vi "Set SubPanel Controls Values.vi"(7 "Subpanels Map":map{string, refnum<vi>}(c390), 8 "error in (no error)":errorcluster, 11 "Schedule Block in":refnum<class "Schedule Block.lvclass">) -> (0 "error out":errorcluster, 2 "SBlock Type":string, 3 "SubPanel VI out":refnum<vi>)   [LabVIEW 2020, in "CIRCUS_uServices.lvlib" / "Scheduler.lvlib" / "Scheduler.lvclass"]
uses:
  Scheduler.lvclass
  Run Utilities/Schedule Block/Schedule Block.lvclass
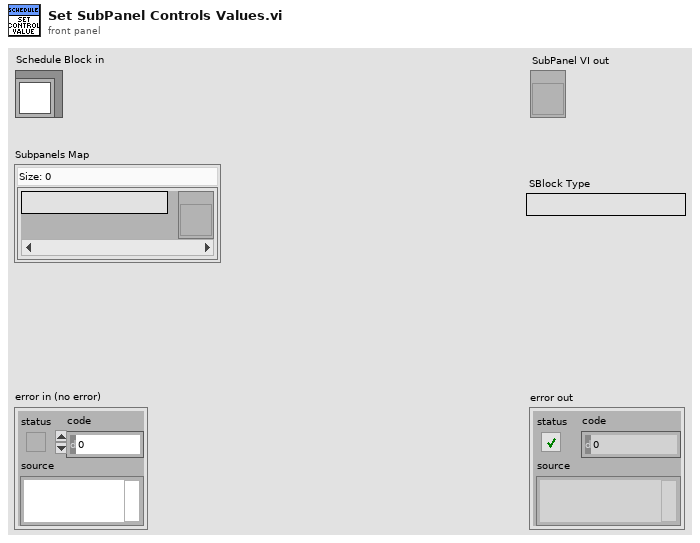
[diagram p1: front panel]
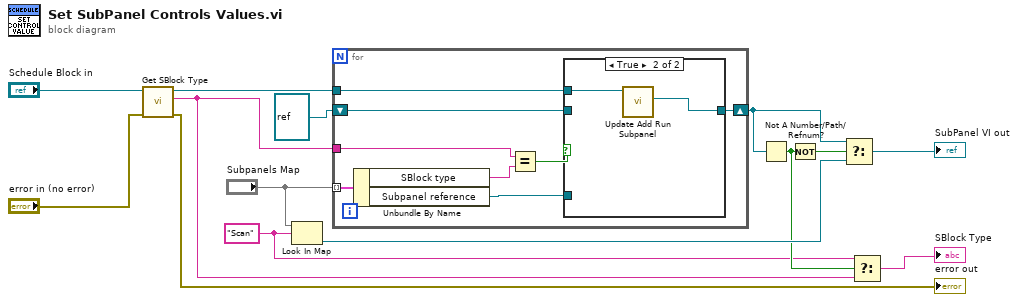
[diagram p0: block diagram]
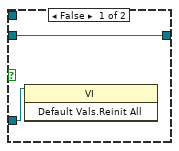
[diagram p2: hidden frame]
diagram:
  w2 = "Scan" ("f")
  n1 = call-dynamic "Get SBlock Type.vi"("error in (no error)"="error in (no error)", "Schedule Block in"="Schedule Block in") -> ("error out"=→"error out":errorcluster, "SBlock Type"=w3:string, "Schedule Block out"=w10:refnum<class "Schedule Block.lvclass">)  [unwired: 7 in]
  n2 = Look In Map(map="Subpanels Map", key=w2) -> (value=w6:refnum<vi>)  [unwired: 1 in, 1 out]
  n3 = for {
    tunnel: w10 -> [w18]
    tunnel: w3 -> [w21]
    tunnel: "Subpanels Map" -> [w22] mode=indexing
    shift-right: [w17] -> w7
    shift-left: refnum<vi> refnum ("y") -> [w16]
    n4 = Unbundle By Name(w22) -> ("SBlock type"=w20:string, "Subpanel reference"=w15:refnum<vi>)
    n5 = Equal?(x=w21, y=w20) -> (x = y?=w19:bool)
    n6 = case shown="True" w19 {
      tunnel: w18 -> [_ w26]
      tunnel: [w24 w25] -> w17
      tunnel: w16 -> [w24 _]
      tunnel: w15 -> [w23 _]
      frame False {
        n7 = invoke class="VI" method="Default Vals.Reinit All"(reference=w23) -> ()  [unwired: 2 in, 3 out]
      }
      frame True {
        n8 = call-dynamic "Update Add Run Subpanel.vi"("Schedule Block in"=w26) -> ("Subpanel ref"=w25:refnum<vi>)  [unwired: 8 in, 2 out]
      }
    }
  }
  n9 = Not A Number/Path/Refnum?(number/path/refnum=w7) -> (NaN/Path/Refnum?=w4:bool)
  n10 = Not(x=w4) -> (.not. x?=w5:bool)
  n11 = Select(t=w7, s=w5, f=w6) -> (s? t:f=→"SubPanel VI out":refnum<vi>)
  n12 = Select(t=w2, s=w4, f=w3) -> (s? t:f=→"SBlock Type":string)
